vi "Fire Quit Event.vi"(8 "error in (no error)":errorcluster, 10 "Force Quit?":bool, 11 "ConfirmQuitSpecPage in":refnum<class "ConfirmQuitSpecPage.lvclass">) -> (0 "error out":errorcluster, 2 "Quit OK?":bool, 3 "ConfirmQuitSpecPage out":refnum<class "ConfirmQuitSpecPage.lvclass">)   [LabVIEW 2016, in "ConfirmQuitSpecPage.lvclass"]
uses:
  <resource>/dialog/NewProjectWizard/SpecPage/ConfirmQuitSpecPage/ConfirmQuitSpecPage.lvclass
  <resource>/dialog/NewProjectWizard/SpecPage/ConfirmQuitSpecPage/ConfirmQuitSpecPage.lvclass/ConfirmQuitSpecPage.ctl
panel:
  # "In the ConfirmQuit spec pages, the Force Quit? is used by the framework to notify the Spec Page whether it is allowed to abort the quit or not.  If Force Quit? is true, the Spec Page should\nquit, without doing any verification or prompting.  This happens if the user Cancels the wizard, or if a user goes Back/Next and\na different Spec Page is loaded.  We need a way to force a quit to occur.  Force Quit? is false when it is a normal \"Finish\" from the wizard.  It gives the Spec Page an opportunity to do\nverification and tell the framework whether the Quit is allowed\nor not."
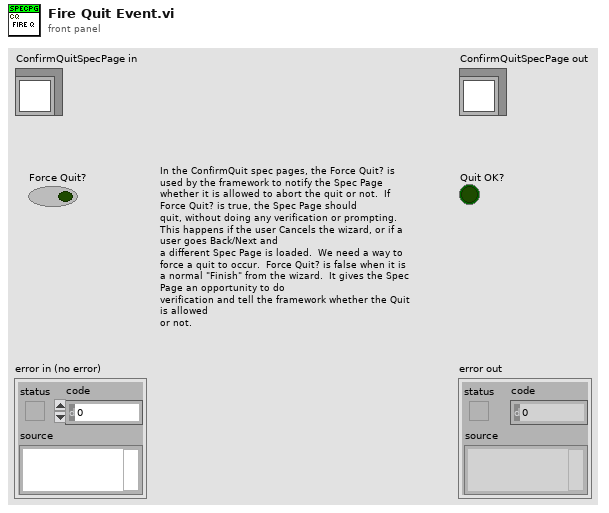
[diagram p1: front panel]
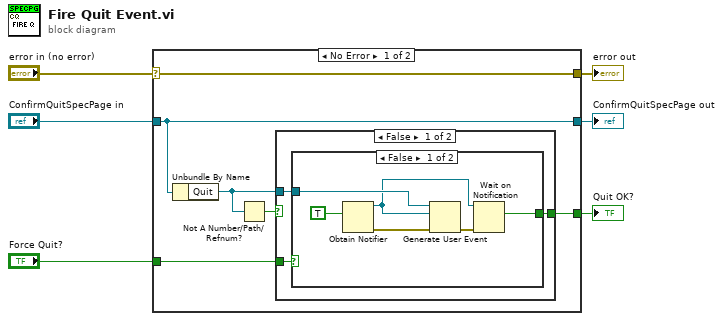
[diagram p0: block diagram]
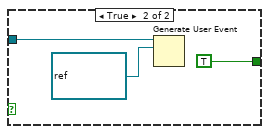
[diagram p2: hidden frame]
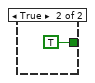
[diagram p3: hidden frame]
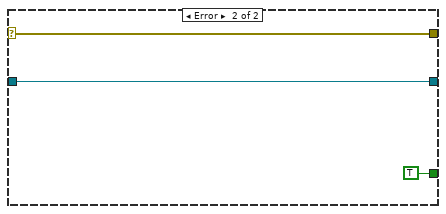
[diagram p4: hidden frame]
diagram:
  n1 = case shown="No Error" "error in (no error)" {
    selector: "error in (no error)" -> [w8 w28]
    tunnel: [w8 w28] -> w5
    tunnel: [w12 w27] -> w3
    tunnel: "ConfirmQuitSpecPage in" -> [w12 w27]
    tunnel: [w9 TRUE] -> w2
    tunnel: "Force Quit?" -> [w7 _]
    frame No Error {
      n2 = Unbundle By Name(w12) -> ("Quit"=w10:refnum<user-event>)
      n3 = Not A Number/Path/Refnum?(number/path/refnum=w10) -> (NaN/Path/Refnum?=w11:bool)
      n4 = case shown="False" w11 {
        tunnel: w10 -> [w15 _]
        tunnel: [w14 TRUE] -> w9
        tunnel: w7 -> [w13 _]
        frame False {
          n5 = case shown="False" w13 {
            tunnel: w15 -> [w20 w24]
            tunnel: [w16 TRUE] -> w14
            frame False {
              n6 = Obtain Notifier(notification data type=TRUE) -> (notifier out=w17:refnum<notifier>, error out=w19:errorcluster)  [unwired: 3 in, 1 out]
              n7 = Generate User Event(user event=w20, event data cluster=w17, error in=w19) -> (error out=w18:errorcluster)  [unwired: 1 in, 1 out]
              n8 = Wait on Notification(notifier=w17, error in (no error)=w18) -> (notification=w16:bool)  [unwired: 2 in, 3 out]
            }
            frame True {
              n9 = Generate User Event(user event=w24, event data cluster=refnum<notifier> refnum ("event data")) -> ()  [unwired: 2 in, 2 out]
            }
          }
        }
        frame True {
        }
      }
    }
    frame Error {
    }
  }
  "error out" <- w5
  "ConfirmQuitSpecPage out" <- w3
  "Quit OK?" <- w2
